vi "总氮固定站质控流程.vi"(6 "队列输入TN":refnum<queue>, 9 "总氮":bool, 10 "总氮量程切换":enum32{"H", "L", "AUTO"}(ring)=enum."AUTO") -> (3 "布尔":bool)   [LabVIEW 2016, in "质控单元.lvlib"]
panel:
  out "参数 out":T1
  out "总氮中断报警":bool
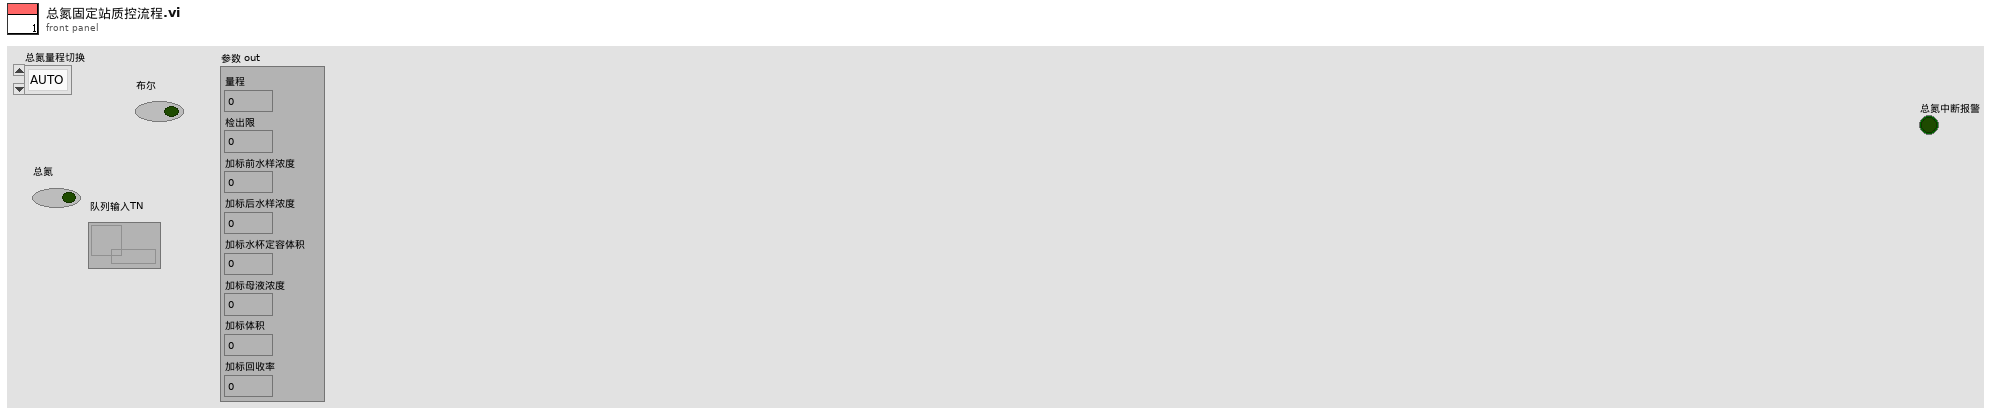
[diagram p1: front panel]
types:
  T1 = cluster{"量程":dbl, "检出限":dbl, "加标前水样浓度":dbl, "加标后水样浓度":dbl, "加标水杯定容体积":dbl, "加标母液浓度":dbl, "加标体积":dbl, "加标回收率":dbl}
  T2 = enum16{"待机", "启动氨氮水样", "氨氮测量中", "启动氨氮加标", "启动氨氮加标回收", "氨氮加标回收测量中", "启动总氮水样", "总氮测量中", "启动总氮加标", "启动总氮加标回收", "总氮加标回收测量中", "启动总磷水样", "总磷水样测量中", "启动总磷加标", "启动总磷加标回收", "总磷加标回收测量中", "结束"}
  T3 = cluster{"站号":u16, "量程切换":enum32{"H", "L", "AUTO"}, "控制命令":enum16{"启动测量", "标样核查", "零点核查", "跨度核查", "空白测试", "平行样测试", "加标回收", "空白校准", "标样校准", "初始化（清洗）", "停止测试", "仪器重启", "校时", "模式设置", "测量间隔设置"}, "模式设置":enum16{"待机", "连续模式", "周期模式", "定点模式", "受控模式", "手动模式"}, "测量间隔":u16}
  T4 = cluster{"时间标识":timestamp, "设备":string, "日志信息":string}
  T5 = cluster{"系统时间":timestamp, "工作状态":enum16{"空闲", "水样测试", "标样核查", "零点核查", "跨度核查", "空白测试", "平行样测试", "加标回收", "空白校准", "标样校准", "初始化（清洗）"}, "测量模式":enum16{"待机", "连续模式", "周期模式", "定点模式", "受控模式", "手动模式"}, "告警代码":enum16{"无告警", "缺试剂告警", "缺水样告警", "缺蒸馏水告警", "缺标液告警", "仪表漏液告警", "标定异常告警", "超量程告警", "加热异常", "低试剂预警", "超上限告警", "超下限告警", "仪表内部其他异常", "滴定异常告警", "电极异常告警", "量程切换告警", "参数设置告警", "PH电极电位异常", "电导率电极异常", "浊度光度异常", "溶解氧电极异常", "溶解氧光强异常", "温度异常告警", "PH异常告警", "溶解氧异常告警", "电导率异常告警", "浊度异常告警", "叶绿素异常告警", "藻密度异常告警", "蓝绿藻异常告警", "ORP异常告警", "氨氮异常告警", "清洁刷异常告警", "SD卡异常告警", "蓝牙异常告警", "Wifi异常告警", "流程异常告警"}, "故障代码":enum16{"无故障", "电机故障", "温度故障", "通讯故障", "滴定故障"}, "日志代码":u16, "软件版本":u16, "F0":sgl, "F1":sgl, "F2":sgl, "F3":sgl, "T":sgl, "H":sgl, "id":u16, "flowid":u16, "量程":u16, "总磷控温温度1":sgl, "营养盐控温温度2":sgl, "ADC":sgl}
  T6 = enum16{"空闲", "水样测试", "标样核查", "零点核查", "跨度核查", "空白测试", "平行样测试", "加标回收", "空白校准", "标样校准", "初始化（清洗）"}
  T7 = cluster{"因子编码":u32, "单位":u16, "标样参考值":sgl, "水样数据时间":timestamp, "水样实测值":sgl, "水样数据标识":string, "标样数据时间":timestamp, "标样实测值":sgl, "标样数据标识":string, "空白数据时间":timestamp, "空白实测值":sgl, "空白数据标识":string, "零点核查数据时间":timestamp, "零点核查实测值":sgl, "零点核查数据标识":string, "跨度核查数据时间":timestamp, "跨度核查实测值":sgl, "跨度核查数据标识":string, "加标回收数据时间":timestamp, "加标回收实测值":sgl, "加标回收数据标识":string, "平行样数据时间":timestamp, "平行样实测值":sgl, "平行样数据标识":string}
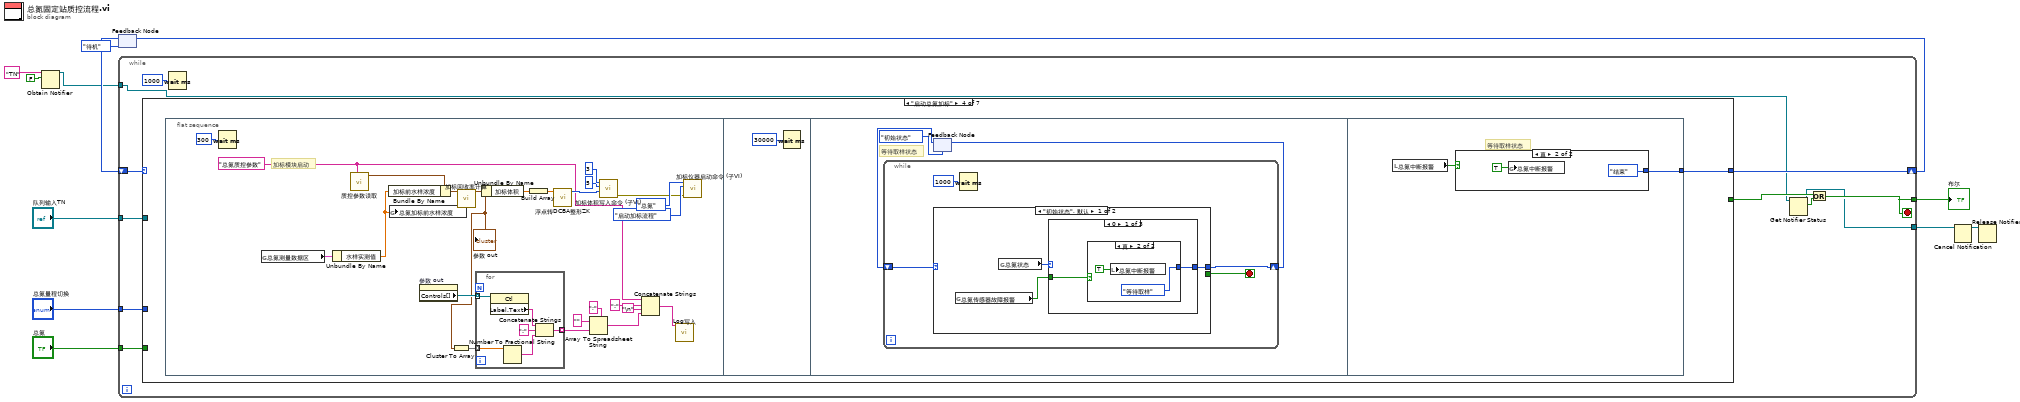
[diagram p0: block diagram]
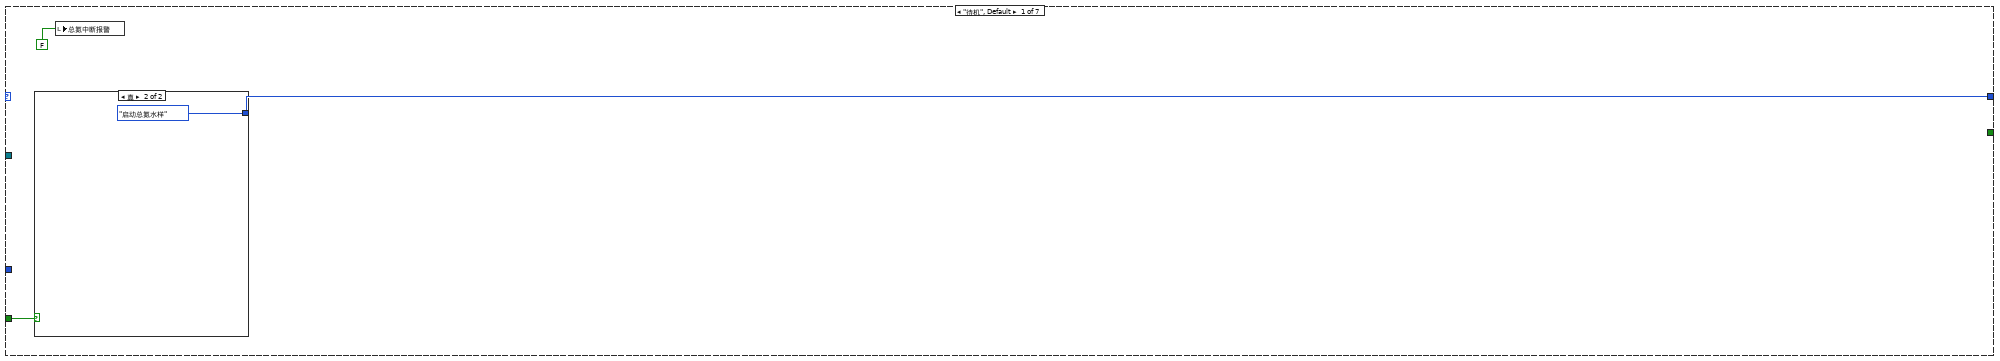
[diagram p2: hidden frame]
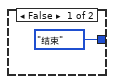
[diagram p3: hidden frame]
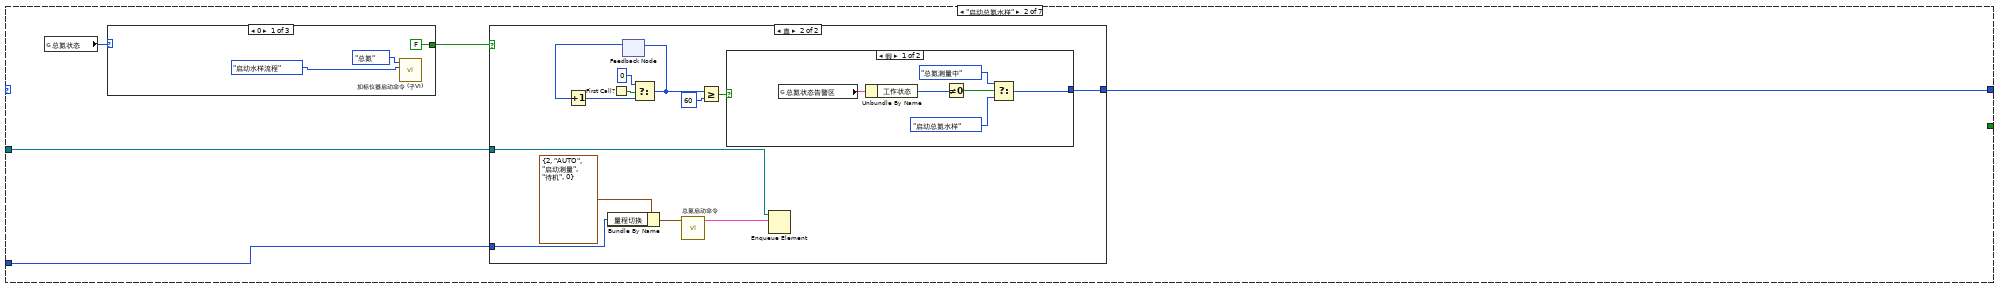
[diagram p4: hidden frame]
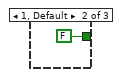
[diagram p5: hidden frame]
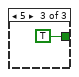
[diagram p6: hidden frame]
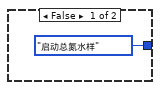
[diagram p7: hidden frame]
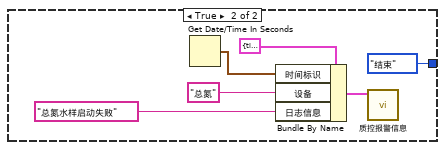
[diagram p8: hidden frame]
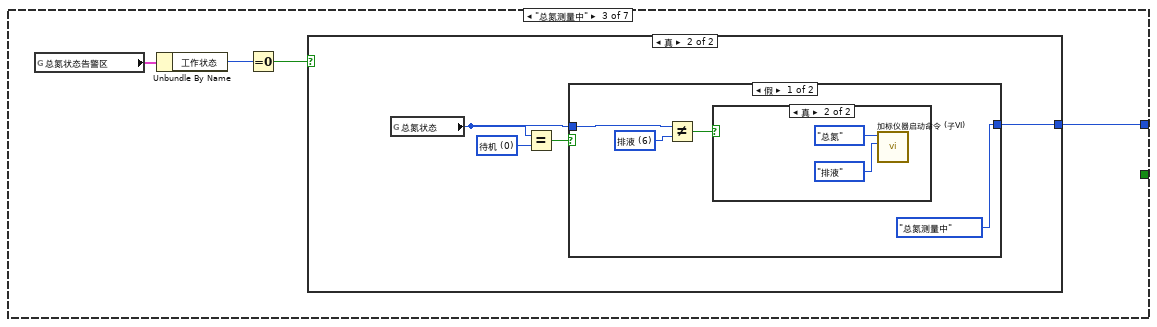
[diagram p9: hidden frame]
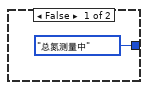
[diagram p10: hidden frame]
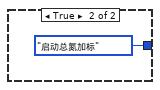
[diagram p12: hidden frame]
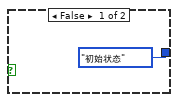
[diagram p13: hidden frame]
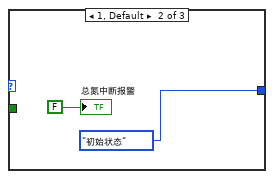
[diagram p14: hidden frame]
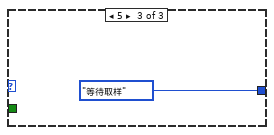
[diagram p15: hidden frame]
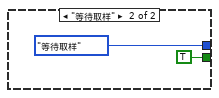
[diagram p16: hidden frame]
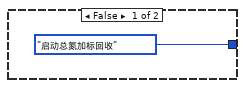
[diagram p17: hidden frame]
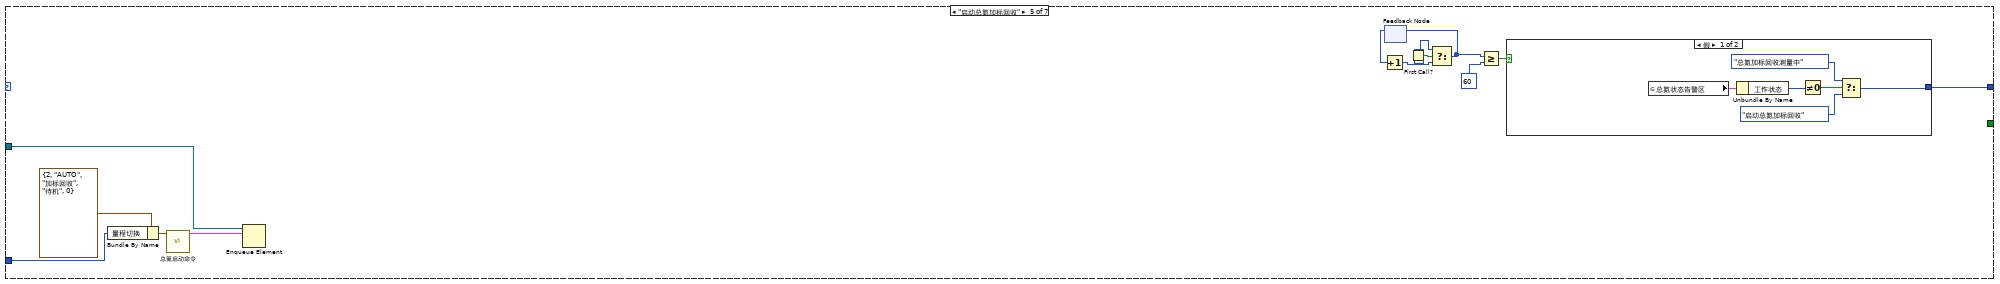
[diagram p18: hidden frame]
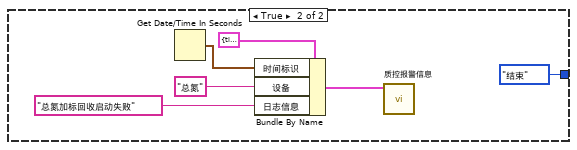
[diagram p19: hidden frame]
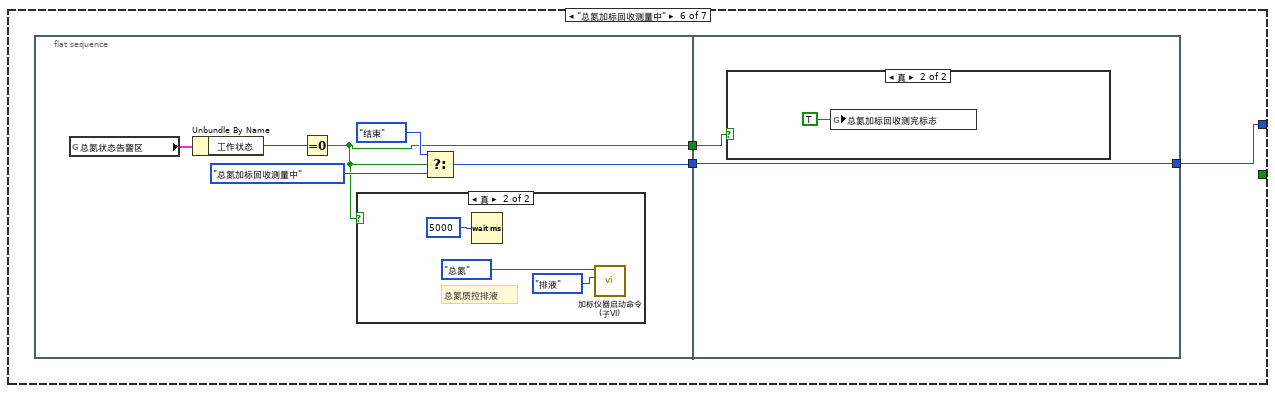
[diagram p20: hidden frame]
diagram:
  n1 = Obtain Notifier(name (unnamed)="TN" ("名称（未命名）"), notification data type=FALSE) -> (notifier out=w3:refnum<notifier>)  [unwired: 2 in, 2 out]
  n2 = feedback #1(T2."待机") -> (w6:T2)
  n3 = while {
    tunnel: "队列输入TN" -> [w21]
    tunnel: "总氮量程切换" -> [w20]
    tunnel: "总氮" -> [w23]
    tunnel: [w15] -> w11
    shift-right: [w22] -> w9
    shift-left: w6 -> [w19]
    tunnel: w3 -> [w14]
    tunnel: [w13] -> w1
    stop <- w15 stop-if-true
    n4 = case shown="\"启动总氮加标\"" w19 {
      tunnel: [w26 w33 w65 w81 w143 w164 T2."结束"] -> w22
      tunnel: [_ _ _ _ _ _ TRUE] -> w16
      tunnel: w23 -> [w25 _ _ _ _ _ _]
      tunnel: w21 -> [_ w32 _ _ w142 _ _]
      tunnel: w20 -> [_ w31 _ _ w139 _ _]
      frame "待机", Default {
        n5 = case shown="真" w25 {
          tunnel: [T2."结束" T2."启动总氮水样"] -> w26
          frame False {
          }
          frame True {
          }
        }
        n6 = local write "总氮中断报警"(FALSE ("氨氮中断报警")) -> ()
      }
      frame "启动总氮水样" {
        n7 = global read "加标回收状态全局变量.vi" "总氮状态"() -> (w30:u16)
        n8 = case shown="0" w30 {
          tunnel: [FALSE ("s") FALSE ("s") TRUE ("s")] -> w29
          frame 0 {
            n9 = call "加标仪器启动命令 (子VI).vi"("启动命令"=enum16{"启动水样流程", "启动加标流程", "排液", "停止"}."启动水样流程", "仪器"=enum16{"", "氨氮", "总磷", "总氮", "CODMn", "CODCr"}."总氮") -> ()  [unwired: 9 in, 1 out]
          }
          frame 1, Default {
          }
          frame 5 {
          }
        }
        n10 = case shown="真" w29 {
          tunnel: [T2."启动总氮水样" w52] -> w33
          tunnel: w32 -> [_ w44]
          tunnel: w31 -> [_ w41]
          frame False {
          }
          frame True {
            n11 = Bundle By Name(cluster=T3 {"站号"=2, "量程切换"=enum."AUTO", "控制命令"=enum."启动测量", "模式设置"=enum."待机", "测量间隔"=0} ("参数"), "量程切换"=w41) -> (w43:T3)
            n12 = First Call?() -> (First Call?: T/F=w50:bool)
            n13 = feedback #2() -> (w49:i32)  [unwired: 1 in]
            n14 = Increment(x=w49) -> (x+1=w48:i32)
            n15 = Select(t=0, s=w50, f=w48) -> (s? t:f=w47:i32)
            n16 = feedback-in #2(w47) -> ()
            n17 = call "总氮启动命令.vi"("参数"=w43) -> ("启动命令"=w40:cluster{"命令":string, "data":variant})  [unwired: 10 in]
            n18 = Greater Or Equal?(x=w47, y=60) -> (x >= y?=w45:bool)
            n19 = case shown="假" w45 {
              tunnel: [w57 T2."结束"] -> w52
              frame False {
                n20 = global read "与总氮交互全局.vi" "总氮状态告警区"() -> (w54:T5)
                n21 = Unbundle By Name(w54) -> ("工作状态"=w53:T6)
                n22 = Not Equal To 0?(x=w53) -> (x != 0?=w58:bool)
                n23 = Select(t=T2."总氮测量中", s=w58, f=T2."启动总氮水样") -> (s? t:f=w57:T2)
              }
              frame True {
                n24 = Get Date/Time In Seconds() -> (seconds since 1Jan1904=w64:timestamp)
                n25 = Bundle By Name(cluster=T4 {"时间标识"=timestamp(0 s since 1904-01-01), "设备"="", "日志信息"=""} ("data in"), "时间标识"=w64, "设备"="总氮", "日志信息"="总氮水样启动失败") -> (w59:T4)
                n26 = call "质控报警信息.vi"("data in"=w59) -> ()  [unwired: 10 in, 1 out]
              }
            }
            n27 = Enqueue Element(queue=w44, element=w40) -> ()  [unwired: 2 in, 3 out]
          }
        }
      }
      frame "总氮测量中" {
        n28 = global read "与总氮交互全局.vi" "总氮状态告警区"() -> (w68:T5)
        n29 = Unbundle By Name(w68) -> ("工作状态"=w66:T6)
        n30 = Equal To 0?(x=w66) -> (x = 0?=w67:bool)
        n31 = case shown="真" w67 {
          tunnel: [T2."总氮测量中" w71] -> w65
          frame False {
          }
          frame True {
            w73 = u16 0 items=["待机", "润洗", "进样", "进样完成", "柱塞泵加标", "等待取液", "排液"] ("氨氮状态")
            n32 = global read "加标回收状态全局变量.vi" "总氮状态"() -> (w70:u16)
            n33 = Equal?(x=w70, y=w73) -> (x = y?=w72:bool)
            n34 = case shown="假" w72 {
              tunnel: [T2."总氮测量中" T2."启动总氮加标"] -> w71
              tunnel: w70 -> [w74 _]
              frame False {
                w76 = u16 6 items=["待机", "润洗", "进样", "进样完成", "柱塞泵加标", "等待取液", "排液"] ("氨氮状态")
                n35 = Not Equal?(x=w74, y=w76) -> (x != y?=w75:bool)
                n36 = case shown="真" w75 {
                  frame False {
                  }
                  frame True {
                    n37 = call "加标仪器启动命令 (子VI).vi"("启动命令"=enum16{"启动水样流程", "启动加标流程", "排液", "停止"}."排液", "仪器"=enum16{"", "氨氮", "总磷", "总氮", "CODMn", "CODCr"}."总氮") -> ()  [unwired: 9 in, 1 out]
                  }
                }
              }
              frame True {
              }
            }
          }
        }
      }
      frame "启动总氮加标" {
        n38 = flat-sequence {
          tunnel: [w134] -> w81
          frame #0 {
            w83 = "总氮质控参数" ("section")
            # "加标模块启动"
            n39 = Wait (ms)(milliseconds to wait=u32 300 ("等待时间（毫秒）")) -> ()  [unwired: 1 out]
            n40 = global read "与总氮交互全局.vi" "总氮测量数据区"() -> (w100:T7)
            n41 = Unbundle By Name(w100) -> ("水样实测值"=w102:sgl)
            n42 = call "质控参数读取.vi"("section"=w83) -> ("参数"=w104:T1)  [unwired: 9 in, 1 out]
            n43 = Bundle By Name(cluster=w104, "加标前水样浓度"=w102) -> (w105:T1)
            n44 = global write "水样浓度全局.vi" "总氮加标前水样浓度"(w102) -> ()
            n45 = property on="参数 out" class="Clust (严格)"() -> ("Controls[]"=w88:refnum<vi>[])  [unwired: 2 in, 2 out]
            n46 = call "加标回收率计算.vi"("参数"=w105) -> ("参数 out"=w87:T1)  [unwired: 9 in, 1 out]
            "参数 out" <- w87
            n47 = Cluster To Array(cluster=w87) -> (array=w90:dbl[])
            n48 = for {
              tunnel: w88 -> [w111] mode=indexing
              tunnel: w90 -> [w109] mode=indexing
              tunnel: [w106] -> w89 mode=indexing
              n49 = property class="Ctl"(reference=w111) -> ("Label.Text"=w110:string)  [unwired: 1 in, 2 out]
              n50 = Number To Fractional String(number=w109) -> (F-format string=w107:string)  [unwired: 3 in]
              n51 = Concatenate Strings(w110, ":" ("字符串"), w107) -> (w106:string)
            }
            n52 = Unbundle By Name(w87) -> ("加标体积"=w103:dbl)
            n53 = Build Array(w103) -> (w99:dbl[])
            n54 = call "浮点转DCBA整形ZK.vi"("浮点数"=w99) -> ("DCBA整形输出"=w94:u16[])  [unwired: 10 in]
            n55 = Array To Spreadsheet String(delimiter (Tab)=";" ("分隔符(Tab)"), array=w89, 3:"") -> (spreadsheet string=w85:string)
            n56 = call "加标体积写入命令 (子VI).vi"("values"=w94, "starting address"=u16 5, "Slave ID"=u16 3 ("value")) -> ("错误输出"=w93:errorcluster)  [unwired: 8 in]
            n57 = Concatenate Strings(w83, ":" ("字符串"), "\n", w85) -> (w82:string)
            n58 = call "Log写入.vi"("Log"=w82) -> ()  [unwired: 11 in]
            n59 = call "加标仪器启动命令 (子VI).vi"("错误输入（无错误）"=w93, "启动命令"=enum16{"启动水样流程", "启动加标流程", "排液", "停止"}."启动加标流程", "仪器"=enum16{"", "氨氮", "总磷", "总氮", "CODMn", "CODCr"}."总氮") -> ()  [unwired: 8 in, 1 out]
          }
          frame #1 {
            n60 = Wait (ms)(milliseconds to wait=u32 30000 ("等待时间（毫秒）")) -> ()  [unwired: 1 out]
          }
          frame #2 {
            # "等待取样状态"
            n61 = feedback #3(enum16{"初始状态", "等待取样"}."初始状态") -> (w114:enum16{"初始状态", "等待取样"})
            n62 = while {
              shift-right: [w118] -> w115
              shift-left: w114 -> [w119]
              stop <- w117 stop-if-true
              n63 = case shown="\"初始状态\", 默认" w119 {
                tunnel: [w122 enum16{"初始状态", "等待取样"}."等待取样"] -> w118
                tunnel: [_ TRUE] -> w117
                frame "初始状态", Default {
                  n64 = global read "质控中断报警全局.vi" "总氮传感器故障报警"() -> (w120:bool)
                  n65 = global read "加标回收状态全局变量.vi" "总氮状态"() -> (w121:u16)
                  n66 = case shown="0" w121 {
                    tunnel: [w124 enum16{"初始状态", "等待取样"}."初始状态" enum16{"初始状态", "等待取样"}."等待取样"] -> w122
                    tunnel: w120 -> [w123 _ _]
                    frame 0 {
                      n67 = case shown="真" w123 {
                        tunnel: [enum16{"初始状态", "等待取样"}."初始状态" enum16{"初始状态", "等待取样"}."等待取样"] -> w124
                        frame False {
                        }
                        frame True {
                          n68 = local write "总氮中断报警"(TRUE ("氨氮中断报警")) -> ()
                        }
                      }
                    }
                    frame 1, Default {
                      "总氮中断报警" <- FALSE ("总氮中断报警")
                    }
                    frame 5 {
                    }
                  }
                }
                frame "等待取样" {
                }
              }
              n69 = Wait (ms)(milliseconds to wait=u32 1000 ("等待时间（毫秒）")) -> ()  [unwired: 1 out]
            }
            n70 = feedback-in #3(w115) -> ()
          }
          frame #3 {
            # "等待取样状态"
            n71 = local read "总氮中断报警"() -> (w133:bool)
            n72 = case shown="真" w133 {
              tunnel: [T2."启动总氮加标回收" T2."结束"] -> w134
              frame False {
              }
              frame True {
                n73 = global write "质控中断报警全局.vi" "总氮中断报警"(TRUE ("总氮中断报警")) -> ()
              }
            }
          }
        }
      }
      frame "启动总氮加标回收" {
        n74 = Bundle By Name(cluster=T3 {"站号"=2, "量程切换"=enum."AUTO", "控制命令"=enum."加标回收", "模式设置"=enum."待机", "测量间隔"=0} ("参数"), "量程切换"=w139) -> (w141:T3)
        n75 = call "总氮启动命令.vi"("参数"=w141) -> ("启动命令"=w138:cluster{"命令":string, "data":variant})  [unwired: 10 in]
        n76 = Enqueue Element(queue=w142, element=w138) -> ()  [unwired: 2 in, 3 out]
        n77 = feedback #4() -> (w148:i32)  [unwired: 1 in]
        n78 = Increment(x=w148) -> (x+1=w147:i32)
        n79 = First Call?() -> (First Call?: T/F=w149:bool)
        n80 = Select(t=0, s=w149, f=w147) -> (s? t:f=w146:i32)
        n81 = feedback-in #4(w146) -> ()
        n82 = Greater Or Equal?(x=w146, y=60) -> (x >= y?=w144:bool)
        n83 = case shown="假" w144 {
          tunnel: [w154 T2."结束"] -> w143
          frame False {
            n84 = global read "与总氮交互全局.vi" "总氮状态告警区"() -> (w151:T5)
            n85 = Unbundle By Name(w151) -> ("工作状态"=w156:T6)
            n86 = Not Equal To 0?(x=w156) -> (x != 0?=w155:bool)
            n87 = Select(t=T2."总氮加标回收测量中", s=w155, f=T2."启动总氮加标回收") -> (s? t:f=w154:T2)
          }
          frame True {
            n88 = Get Date/Time In Seconds() -> (seconds since 1Jan1904=w162:timestamp)
            n89 = Bundle By Name(cluster=T4 {"时间标识"=timestamp(0 s since 1904-01-01), "设备"="", "日志信息"=""} ("data in"), "时间标识"=w162, "设备"="总氮", "日志信息"="总氮加标回收启动失败") -> (w157:T4)
            n90 = call "质控报警信息.vi"("data in"=w157) -> ()  [unwired: 10 in, 1 out]
          }
        }
      }
      frame "总氮加标回收测量中" {
        n91 = flat-sequence {
          tunnel: [w170] -> w165
          tunnel: [w166] -> w163
          tunnel: [w176] -> w164
          tunnel: w165 -> [w176]
          tunnel: w163 -> [w175]
          frame #0 {
            n92 = global read "与总氮交互全局.vi" "总氮状态告警区"() -> (w167:T5)
            n93 = Unbundle By Name(w167) -> ("工作状态"=w171:T6)
            n94 = Equal To 0?(x=w171) -> (x = 0?=w166:bool)
            n95 = case shown="真" w166 {
              frame False {
              }
              frame True {
                # "总氮质控排液"
                n96 = Wait (ms)(milliseconds to wait=u32 5000 ("等待时间（毫秒）")) -> ()  [unwired: 1 out]
                n97 = call "加标仪器启动命令 (子VI).vi"("启动命令"=enum16{"启动水样流程", "启动加标流程", "排液", "停止"}."排液", "仪器"=enum16{"", "氨氮", "总磷", "总氮", "CODMn", "CODCr"}."总氮") -> ()  [unwired: 9 in, 1 out]
              }
            }
            n98 = Select(t=T2."结束", s=w166, f=T2."总氮加标回收测量中") -> (s? t:f=w170:T2)
          }
          frame #1 {
            n99 = case shown="真" w175 {
              frame False {
              }
              frame True {
                n100 = global write "质控测完标志全局 1.vi" "总氮加标回收测完标志"(TRUE) -> ()
              }
            }
          }
        }
      }
      frame "结束" {
        n101 = Wait (ms)(milliseconds to wait=u32 5000 ("等待时间（毫秒）")) -> ()  [unwired: 1 out]
      }
    }
    n102 = Wait (ms)(milliseconds to wait=u32 1000 ("等待时间（毫秒）")) -> ()  [unwired: 1 out]
    n103 = Get Notifier Status(notifier=w14) -> (notifier out=w13:refnum<notifier>, current notification=w17:bool)  [unwired: 1 in, 3 out]
    n104 = Or(x=w16, y=w17) -> (x .or. y?=w15:bool)
  }
  "布尔" <- w11
  n105 = feedback-in #1(w9) -> ()
  n106 = Cancel Notification(0:w1) -> (8:w2:refnum<notifier>)  [unwired: 1 in, 2 out]
  n107 = Release Notifier(notifier=w2) -> ()  [unwired: 2 in, 3 out]
